vi "gfitsio-read-column-boolean-1d.vi"(6 "row":i32, 7 "column":string, 8 "error in (no error)":errorcluster, 11 "gfits refnum":T1) -> (0 "error out":errorcluster, 2 "data":bool[](array[boolean]), 3 "dup gfits refnum":T1)   [LabVIEW 2011, in "gfitsio.lvlib"]
doc: "Read elements from an ASCII or binary table column."
uses:
  gfitsio.lvlib
  gfitsio-refnum.ctl
  cfitsio-hdutypes.ctl
  gfitsio.dll
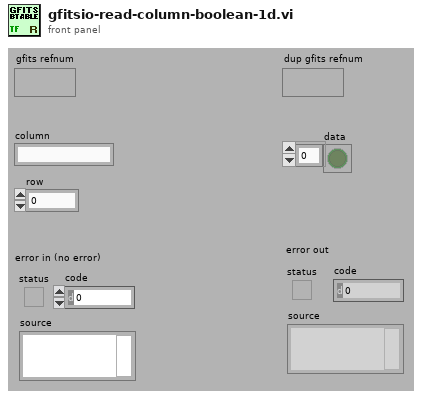
[diagram p1: front panel]
types:
  T1 = typedef "gfitsio.lvlib/gfitsio-refnum.ctl" = refnum<k1>
  T2 = typedef "gfitsio.lvlib/cfitsio-hdutypes.ctl" = i32
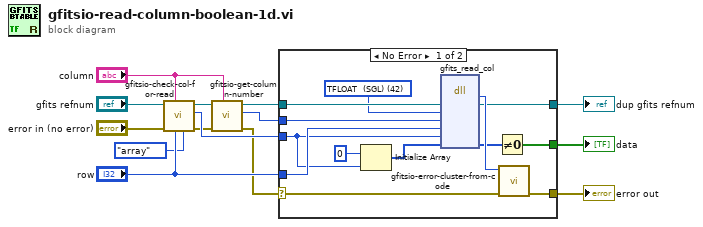
[diagram p0: block diagram]
diagram:
  n1 = call "gfitsio-check-col-for-read.vi"("expected dimensionality"=enum16{"scalar", "array"}."array", "row"="row", "column"="column", "error in (no error)"="error in (no error)", "gfits refnum"="gfits refnum") -> ("error out"=w5:errorcluster, "nelements"=w10:i32, "dup gfits refnum"=w6:T1)  [unwired: 4 in]
  n2 = call "gfitsio-get-column-number.vi"("column"="column", "error in (no error)"=w5, "gfits refnum"=w6) -> ("error out"=w4:errorcluster, "colnum"=w1:i32, "dup gfits refnum"=w3:T1)  [unwired: 6 in]
  n3 = case shown="No Error" w4 {
    selector: w4 -> [w27 w29]
    tunnel: [w26 w29] -> w13
    tunnel: w3 -> [w23 w28]
    tunnel: [w24 w28] -> w9
    tunnel: "row" -> [w21 _]
    tunnel: [w15 _] -> w14
    tunnel: w10 -> [w20 _]
    tunnel: w1 -> [w17 _]
    frame No Error {
      w16 = T2 42 items=["TBIT"=1, "TBYTE  (U8)"=11, "TSBYTE  (I8)"=12, "TLOGICAL"=14, "TSTRING"=16, "TUSHORT  (U16)"=20, "TSHORT  (I16)"=21, "TUINT"=31, "TULONG  (U32)"=40, "TLONG  (I32)"=41, "TFLOAT  (SGL)"=42, "TLONGLONG  (I64)"=81, "TDOUBLE"=82, "TCOMPLEX  (CSG)"=83, "TDOUBLECOMPLEX  (CDB)"=163] ("cfitsio datatype")
      n4 = Initialize Array(0 ("element"), w20) -> (w18:i32[])
      n5 = dll-call lib="C:/BonOMM/BonOMM-SAOMM/SubVIs/gfitsio/gfitsio.dll" fn="gfits_read_col"("dup gfits refnum"=w23, "datatype"=w16, "colnum"=w17, "row"=w21, "nelements"=w20, "data"=w18) -> (w25:i32, "dup gfits refnum"=w24:T1, "data"=w22:i32[])  [unwired: 7 in, 2 out]
      n6 = Not Equal To 0?(x=w22) -> (x != 0?=w15:bool[])
      n7 = call "gfitsio-error-cluster-from-code.vi"("error in (no error)"=w27, "error code"=w25) -> ("error out"=w26:errorcluster)  [unwired: 9 in]
    }
    frame Error {
    }
  }
  "error out" <- w13
  "dup gfits refnum" <- w9
  "data" <- w14
